vi "set Stufentabellen after Reset.vi"(8 "Fehler (Eingang, kein Fehler)":errorcluster, 9 "Komponente in":T3, 10 "Table Index":i32, 11 "Referenzen Cluster":T1) -> (0 "Fehler (Ausgang)":errorcluster, 1 "Komponente out":T3, 2 "EGAK":T2[](array[typedef]), 3 "Stufen Tabellen out":string[][](array[string]))   [LabVIEW 2020]
uses:
  Visualisierungs Elemente/Auswahlfeld.ctl
  Seiten/System Einstellungen V2/Traegergas.ctl
  GD Abfrage Referenzen.ctl
  Aktion Lin Daten aufarbeiten.ctl
  Linearisierung v2.lvlib
  Seiten/System Einstellungen V2/System Einstellungen V2.lvlib
  SpanEinstellungen.lvlib
panel:
  in  "EGAK Array in":string[][](array[string])
  in  "Stufen Tabellen in":string[][][](array[string])
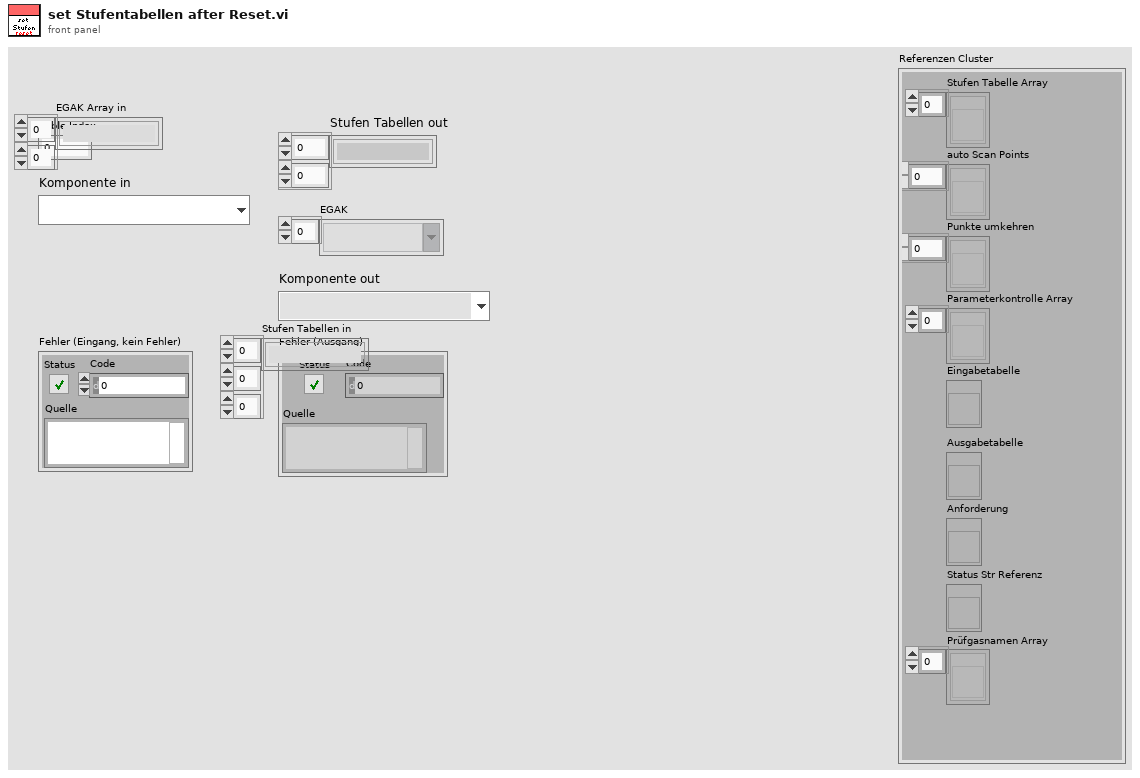
[diagram p1: front panel]
types:
  T1 = typedef "Linearisierung v2.lvlib/SpanEinstellungen.lvlib/GD Abfrage Referenzen.ctl" = cluster{"Stufen Tabelle Array":refnum<vi>[], "auto Scan Points":refnum<vi>[], "Punkte umkehren":refnum<vi>[], "Parameterkontrolle Array":refnum<vi>[], "Eingabetabelle":refnum<vi>, "Ausgabetabelle":refnum<vi>, "Anforderung":refnum<vi>, "Status Str Referenz":refnum<vi>, "Prüfgasnamen Array":refnum<vi>[]}
  T2 = typedef "System Einstellungen V2.lvlib/Traegergas.ctl" = string
  T3 = typedef "Auswahlfeld.ctl" = u16
  T4 = typedef "Linearisierung v2.lvlib/Aktion Lin Daten aufarbeiten.ctl" = enum16{"lesen", "Protkolldaten", "speichern", "laden", "EPA auswerten", "Tabelle schreiben", "Lin auswerten", "Tab init", "Stufentabelle", "EPA aktiviert", "Nachbehandlung laden", "Tabelle löschen", "Istwerte löschen", "Zeile löschen", "Zeile einfügen", "LIN aktiviert", "LIN/EPA aktiv laden", "EGAK Tab", "LIN übernehmen"}
  T5 = typedef "Linearisierung v2.lvlib/Gasteiler.lvlib/Stufen Tabelle.ctl" = string[][]
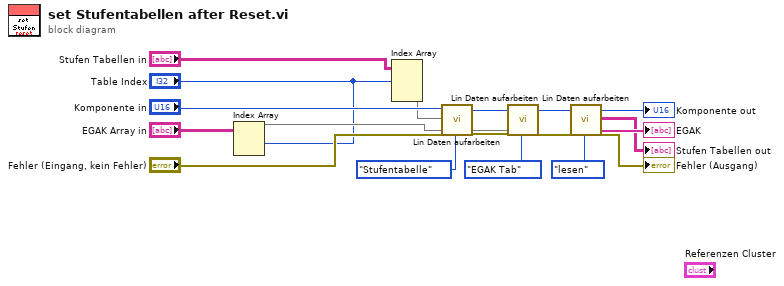
[diagram p0: block diagram]
diagram:
  n1 = Index Array(array="EGAK Array in", index (row)="Table Index") -> (element=w3:string[])  [unwired: 1 in]
  n2 = Index Array(array="Stufen Tabellen in", index (dim 0)="Table Index") -> (element=w13:string[][])  [unwired: 2 in]
  n3 = call "Lin Daten aufarbeiten.vi"("Index (Seite)"="Komponente in", "Stufen Tabelle"=w13, "error in (no error)"="Fehler (Eingang, kein Fehler)", "Aktionen"=Aktion_Lin_Daten_aufarbeiten."Stufentabelle") -> ("Index (Seite) out"=w14:i32, "error out"=w17:errorcluster)  [unwired: 13 in, 9 out]
  n4 = call "Lin Daten aufarbeiten.vi"("Index (Seite)"=w14, "EGAK"=w3, "error in (no error)"=w17, "Aktionen"=Aktion_Lin_Daten_aufarbeiten."EGAK Tab") -> ("Index (Seite) out"=w11:i32, "error out"=w7:errorcluster)  [unwired: 13 in, 9 out]
  n5 = call "Lin Daten aufarbeiten.vi"("Index (Seite)"=w11, "error in (no error)"=w7, "Aktionen"=Aktion_Lin_Daten_aufarbeiten."lesen") -> ("Index (Seite) out"=→"Komponente out":i32, "Stufen Tabelle"=→"Stufen Tabellen out":T5, "EKAG"=→"EGAK":string[], "error out"=→"Fehler (Ausgang)":errorcluster)  [unwired: 14 in, 7 out]
